vi "TCS_Tx_VISA.vi"() -> ()   [LabVIEW 2018]
uses:
  RxTx/RxTx.lvclass
  Serial Communication/Serial Communication.lvclass
panel:
  in  "Serial Communication in":refnum<class "Serial Communication.lvclass">
  in  "RxTx in":refnum<class "RxTx.lvclass">
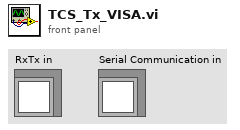
[diagram p1: front panel]
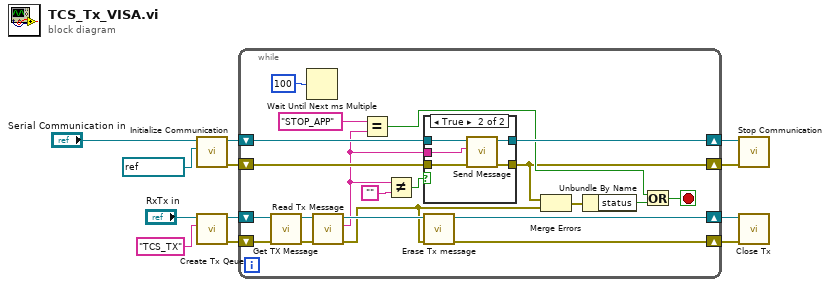
[diagram p0: block diagram]
diagram:
  n1 = call "Initialize Communication.vi"("VISA resource name"=refnum<visa-resource-name> "COM2", "Serial Communication in"="Serial Communication in") -> ("error out"=w3:errorcluster, "Serial Communication out"=w6:refnum<class "Serial Communication.lvclass">)  [unwired: 8 in]
  n2 = call "Create Tx Qeue.vi"("Writer Name"="TCS_TX" ("Reader Name"), "RxTx in"="RxTx in") -> ("error out"=w9:errorcluster, "RxTx out"=w10:refnum<class "RxTx.lvclass">)  [unwired: 8 in]
  n3 = while {
    shift-right: [w14] -> w5
    shift-left: w3 -> [w31]
    shift-right: [w30] -> w4
    shift-left: w6 -> [w32]
    shift-right: [w22] -> w11
    shift-left: w9 -> [w17]
    shift-right: [w23] -> w12
    shift-left: w10 -> [w16]
    stop <- w26 stop-if-true
    n4 = call "Get TX Message.vi"("error in (no error)"=w17, "RxTx in"=w16) -> ("error out"=w18:errorcluster, "RxTx out"=w19:refnum<class "RxTx.lvclass">)  [unwired: 8 in]
    n5 = Wait Until Next ms Multiple(millisecond multiple=u32 100) -> ()  [unwired: 1 out]
    n6 = call "Read Tx Message.vi"("error in (no error)"=w18, "RxTx in"=w19) -> ("error out"=w15:errorcluster, "Tx Message"=w20:string, "RxTx out"=w21:refnum<class "RxTx.lvclass">)  [unwired: 7 in]
    n7 = Equal?(x="STOP_APP", y=w20) -> (x = y?=w28:bool)
    n8 = Not Equal?(x=w20, y="") -> (x != y?=w24:bool)
    n9 = case shown="True" w24 {
      tunnel: w32 -> [w35 w40]
      tunnel: w31 -> [w34 w37]
      tunnel: [w35 w39] -> w30
      tunnel: [w34 w38] -> w14
      tunnel: w20 -> [_ w36]
      frame False {
      }
      frame True {
        n10 = call "Send Message.vi"("error in (no error)"=w37, "Message"=w36, "Serial Communication in"=w40) -> ("error out"=w38:errorcluster, "Serial Communication out"=w39:refnum<class "Serial Communication.lvclass">)  [unwired: 7 in]
      }
    }
    n11 = call "Erase Tx message.vi"("error in (no error)"=w15, "RxTx in"=w21) -> ("error out"=w22:errorcluster, "RxTx out"=w23:refnum<class "RxTx.lvclass">)  [unwired: 8 in]
    n12 = Merge Errors(w14, w15) -> (w33:errorcluster)
    n13 = Unbundle By Name(w33) -> ("status"=w27:bool)
    n14 = Or(x=w28, y=w27) -> (x .or. y?=w26:bool)
  }
  n15 = call "Stop Communication.vi"("error in (no error)"=w5, "Serial Communication in"=w4) -> ()  [unwired: 8 in, 2 out]
  n16 = call "Close Tx.vi"("error in (no error)"=w11, "RxTx in"=w12) -> ()  [unwired: 8 in, 2 out]
